vi "Msgs Output.vi"(11 "TEMPLATE Actor in":refnum<class "TEMPLATE Actor.lvclass">) -> (2 "Msgs":T1)   [LabVIEW 2020, in "_Template.lvlib" / "Templates.lvlib" / "TEMPLATE Actor.lvlib" / "TEMPLATE Actor.lvclass"]
uses:
  TEMPLATE Actor.lvclass
  jettl/jettl/Actor/Actor/Actor.lvclass
  jettl/jettl/Msg/Msg.lvclass
  jettl/jettl/Actor/Msgs.ctl
  jettl/jettl/Actor/Actor.lvlib
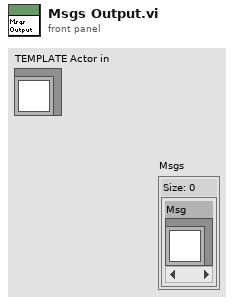
[diagram p1: front panel]
types:
  T1 = typedef "jettl.lvlib/Actor.lvlib/Msgs.ctl" = set{refnum<class "Msg.lvclass">}
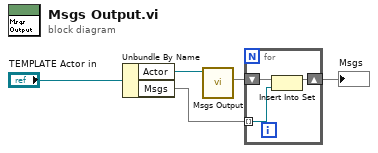
[diagram p0: block diagram]
diagram:
  n1 = Unbundle By Name("TEMPLATE Actor in") -> ("Actor"=w4:refnum<class "Actor.lvclass">, "Msgs"=w2:T1)
  n2 = call-dynamic "Msgs Output.vi"("Get Msgs in"=w4) -> ("Msgs"=w3:T1)  [unwired: 10 in]
  n3 = for {
    tunnel: w2 -> [w7] mode=indexing
    shift-right: [w6] -> w1
    shift-left: w3 -> [w8]
    n4 = Insert Into Set(10:w7, 11:w8) -> (3:w6:T1)  [unwired: 1 out]
  }
  "Msgs" <- w1
